vi "AcquireHardware.vi"(8 "error in (no error)":errorcluster, 11 "Point Grey Camera in":refnum<class "Point Grey Camera.lvclass">) -> (0 "error out":errorcluster, 2 "Image Out":T1(plugin-control), 3 "Point Grey Camera out":refnum<class "Point Grey Camera.lvclass">)   [LabVIEW 2020, in "Point Grey Camera.lvclass"]
uses:
  Point Grey Camera.lvclass
  Point Grey Camera.lvclass/Point Grey Camera.ctl
  NI_Vision_Acquisition_Software.lvlib
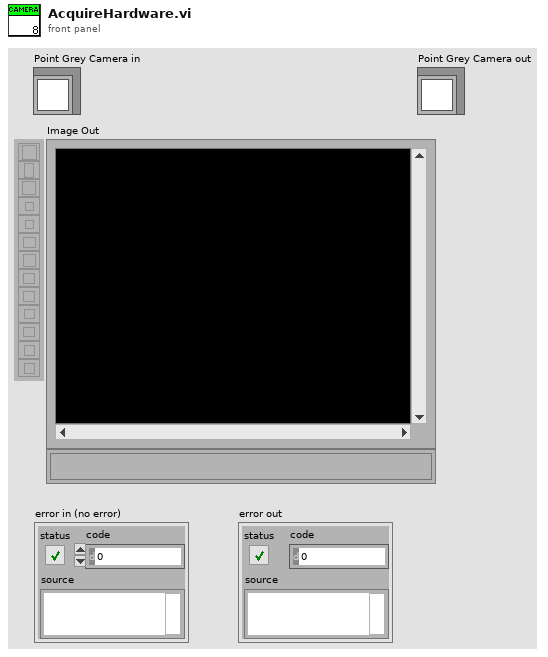
[diagram p1: front panel]
types:
  T1 = typedef "IMAQ Image.ctl" = refnum<image>
  T2 = typedef "IMAQdx.ctl" = refnum<k21>
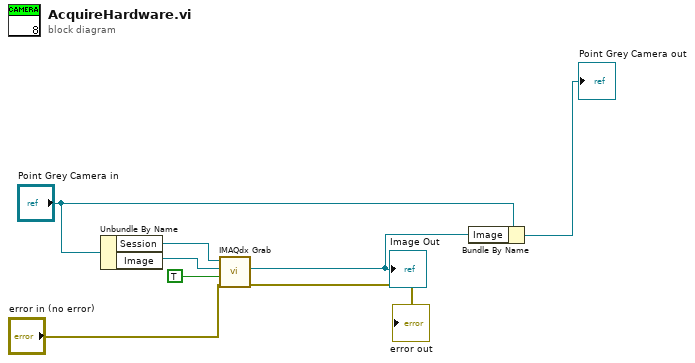
[diagram p0: block diagram]
diagram:
  n1 = Unbundle By Name("Point Grey Camera in") -> ("Session"=w7:T2, "Image"=w8:T1)
  n2 = call "IMAQdx Grab.vi"("error in"="error in (no error)", "Wait for Next Buffer? (Yes)"=TRUE, "Image In"=w8, "Session In"=w7) -> ("error out"=→"error out":errorcluster, "Image Out"=w2:T1)  [unwired: 6 out]
  "Image Out" <- w2
  n3 = Bundle By Name(cluster="Point Grey Camera in", "Image"=w2) -> (→"Point Grey Camera out":refnum<class "Point Grey Camera.lvclass">)
